vi "MultiChannelfFeedbackCooling (FPGA).vi"() -> ()   [LabVIEW 2014]
doc: "This VI will read single point values from 4 channels of a R Series board at a specified rate."
uses:
  <vilib>/rvi/Emulation/niFpgaGetClockAttributes.vi
  <vilib>/rvi/Emulation/niFpgaSctlEmulationGetInTimedLoop.vi
  <vilib>/rvi/Emulation/niFpgaEmulationReportErrorSimple.vi
  <vilib>/rvi/eio/common/nirviEmuTemplateMethod_errors.vi
  <vilib>/rvi/Memory/Memory_Emulation/nirvimemoryFastEmulation.vi
  <vilib>/rvi/Memory/Memory_Emulation/nirvimemoryEmulation.vi
  <vilib>/rvi/Emulation/niFpgaEmulationIsFPGAContextNoSignature.vi
  <vilib>/rvi/DataTransferAndStorage/Container/Common/niFpgaContainerGetUniqueNameForEmu.vi
  <vilib>/rvi/Emulation/niFpgaProcessEmulError.vi
  <vilib>/rvi/errors/nirviReportUnexpectedCaseInternalError (U32).vi
  <vilib>/rvi/Memory/Memory_Emulation/niFpgaMemoryEmulationCacheClearOnFirstRun.vi
  <vilib>/rvi/Memory/Memory_Emulation/nirvimemoryEmulationManagerCache_MakeExclusive.vi
  <vilib>/rvi/Memory/Memory_Emulation/niFpgaMemoryEmulationValidateCache.vi
  <vilib>/rvi/Memory/Memory_Emulation/nirvimemoryEmulationManagerCache_InsertValue.vi
  <vilib>/Utility/error.llb/Clear Errors.vi
  <vilib>/rvi/Memory/Memory_Emulation/nirvimemoryEmulationManagerCache_ReleaseExclusive.vi
  <vilib>/rvi/Memory/Memory_Emulation/nirvimemoryEmulationManagerCache_GetValue.vi
  <vilib>/rvi/Memory/Memory_Emulation/nirvimemoryEmulationManagerCache_SetValue.vi
  <vilib>/rvi/Emulation/niFpgaSctlEmulationResourceMgr.vi
  <vilib>/rvi/Emulation/niFpgaCriticalErrorInLSC.vi
  <vilib>/eio/EIONode/EIONode.xnode
  <vilib>/rvi/DataTransferAndStorage/Container/XNode/niFpgaContainer.xnode
  <vilib>/rvi/FXPMathLib/FxpInterpret/XNode/nifxpmath_Interpret.xnode
panel:
  in  "Piezo Z":i16
  in  "Ref AOM Lvl":i16
  in  "pg_img":fxp<+/-,24,12>
  in  "dg_img":fxp<+/-,24,12>
  in  "ig_img":fxp<+/-,24,6>
  in  "setpt_img":i16
  out "AI_img":i16
  in  "lp coeff_img":i32[](array[numeric])=[1008310688, 32715568]
  in  "Upper lim_img":fxp<+/-,16,16>
  in  "Lower lim_img":fxp<+/-,16,16>
  in  "lp coeff d2":i32[](array[numeric])=[1008310688, 32715568]
  in  "hp coeff_img":i32[](array[numeric])=[946630756, 1010186290]
  out "tot_fb_img":i16
  out "fb_img":i16
  in  "output offset_img":i16
  in  "lp coeff 2":i32[](array[numeric])=[1008310688, 32715568]
  in  "data_buffer3":i16
  in  "Arb gain (ch2)":fxp<+/-,24,12>=0.5 caption="RMS"
  in  "lp coeff 0":i32[](array[numeric])=[1008310688, 32715568]
  in  "lp coeff 1":i32[](array[numeric])=[1008310688, 32715568]
  in  "hp coeff d2":i32[](array[numeric])=[946630756, 1010186290]
  in  "hp coeff 2":i32[](array[numeric])=[946630756, 1010186290]
  in  "hp coeff 1":i32[](array[numeric])=[946630756, 1010186290]
  in  "hp coeff 0":i32[](array[numeric])=[946630756, 1010186290]
  in  "Use_PID2_X 2":bool
  out "AI5":i16
  in  "Dc Pos d2":i16
  out "tot_fb_2":i16
  out "tot_fb_1":i16
  out "tot_fb_0":i16
  out "fb_d2":i16
  in  "output offset 2":i16
  in  "output offset 1":i16
  in  "output offset 0":i16
  in  "Lower lim 4":fxp<+/-,16,16>
  in  "Upper lim d0 3":fxp<+/-,16,16>
  in  "pg d0 3":fxp<+/-,24,12>
  in  "ig d03":fxp<+/-,24,6>
  in  "dg d0 3":fxp<+/-,24,12>
  out "fb_2":i16
  in  "ig 3":fxp<+/-,24,6>
  out "written_address":u32
  in  "ready_to_write":bool
  in  "Arb steps per cycle":u16
  in  "data_buffer2":i16
  in  "data_buffer_1":i16
  in  "write_address":u16
  in  "Arb gain (ch1)":fxp<+/-,24,12>=0.5 caption="RMS"
  in  "Arb gain (ch0)":fxp<+/-,24,12>=0.5 caption="RMS"
  out "fb_1":i16
  out "fb_0":i16
  in  "Dc Pos 1":i16
  in  "Dc Pos 0":i16
  in  "Lower lim 2":fxp<+/-,16,16>
  in  "Upper lim 2":fxp<+/-,16,16>
  in  "dg 2":fxp<+/-,24,12>
  in  "pg 2":fxp<+/-,24,12>
  out "AI2":i16
  in  "Dc Pos 2":i16
  out "AI1":i16
  in  "dg 1":fxp<+/-,24,12>
  in  "Upper lim 1":fxp<+/-,16,16>
  in  "Lower lim 1":fxp<+/-,16,16>
  out "AI0":i16
  in  "dg 0":fxp<+/-,24,12>
  in  "Upper lim 0":fxp<+/-,16,16>
  in  "Lower lim 0":fxp<+/-,16,16>
  in  "Count(uSec)":u32
  out "FPGA Error Out":errorcluster
  in  "Stop":bool
  # "test"
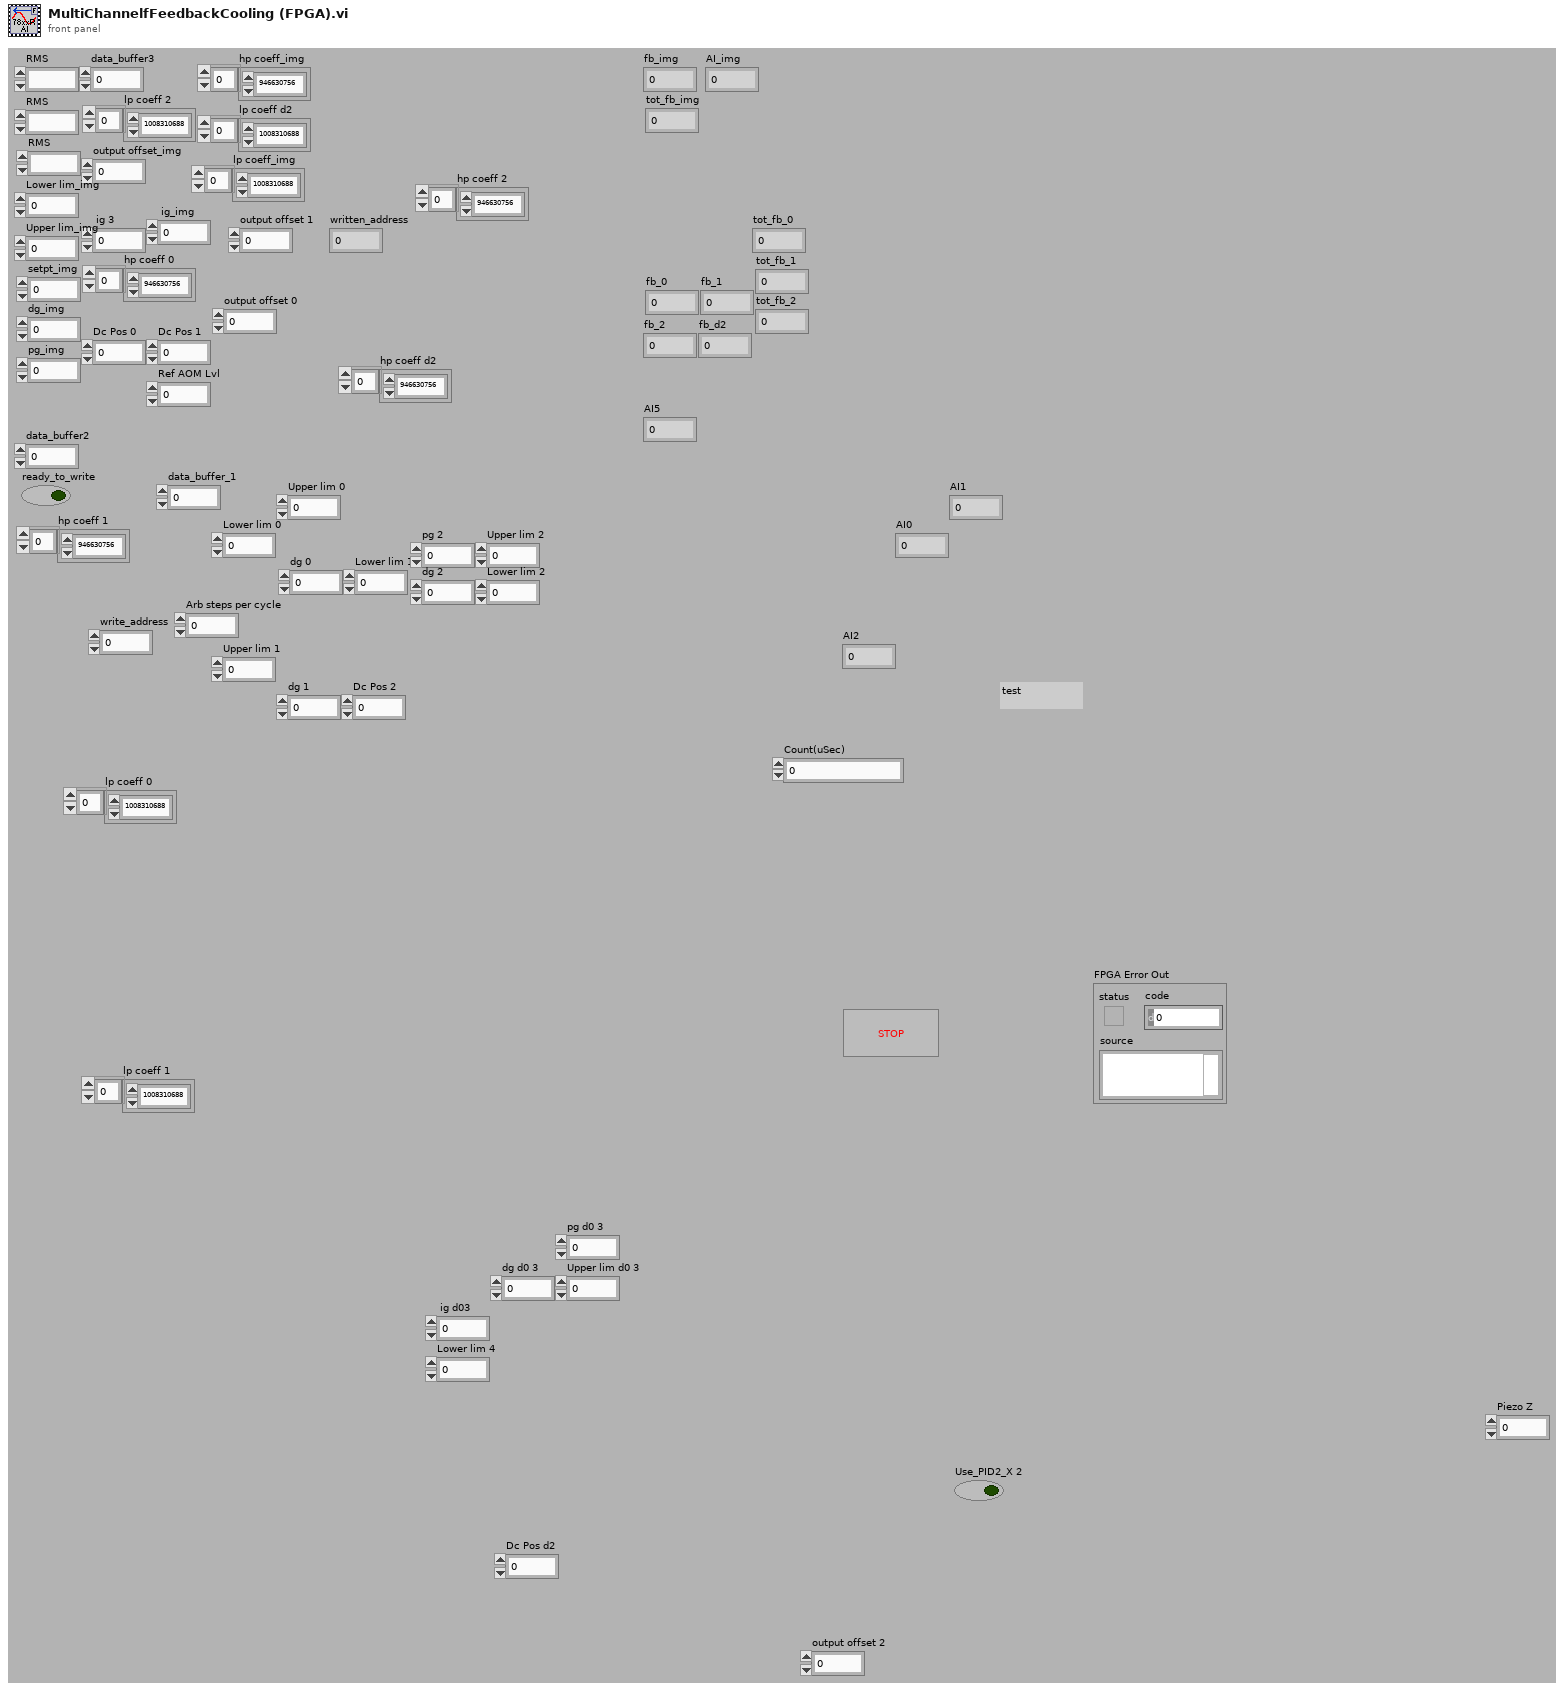
[diagram p1: front panel]
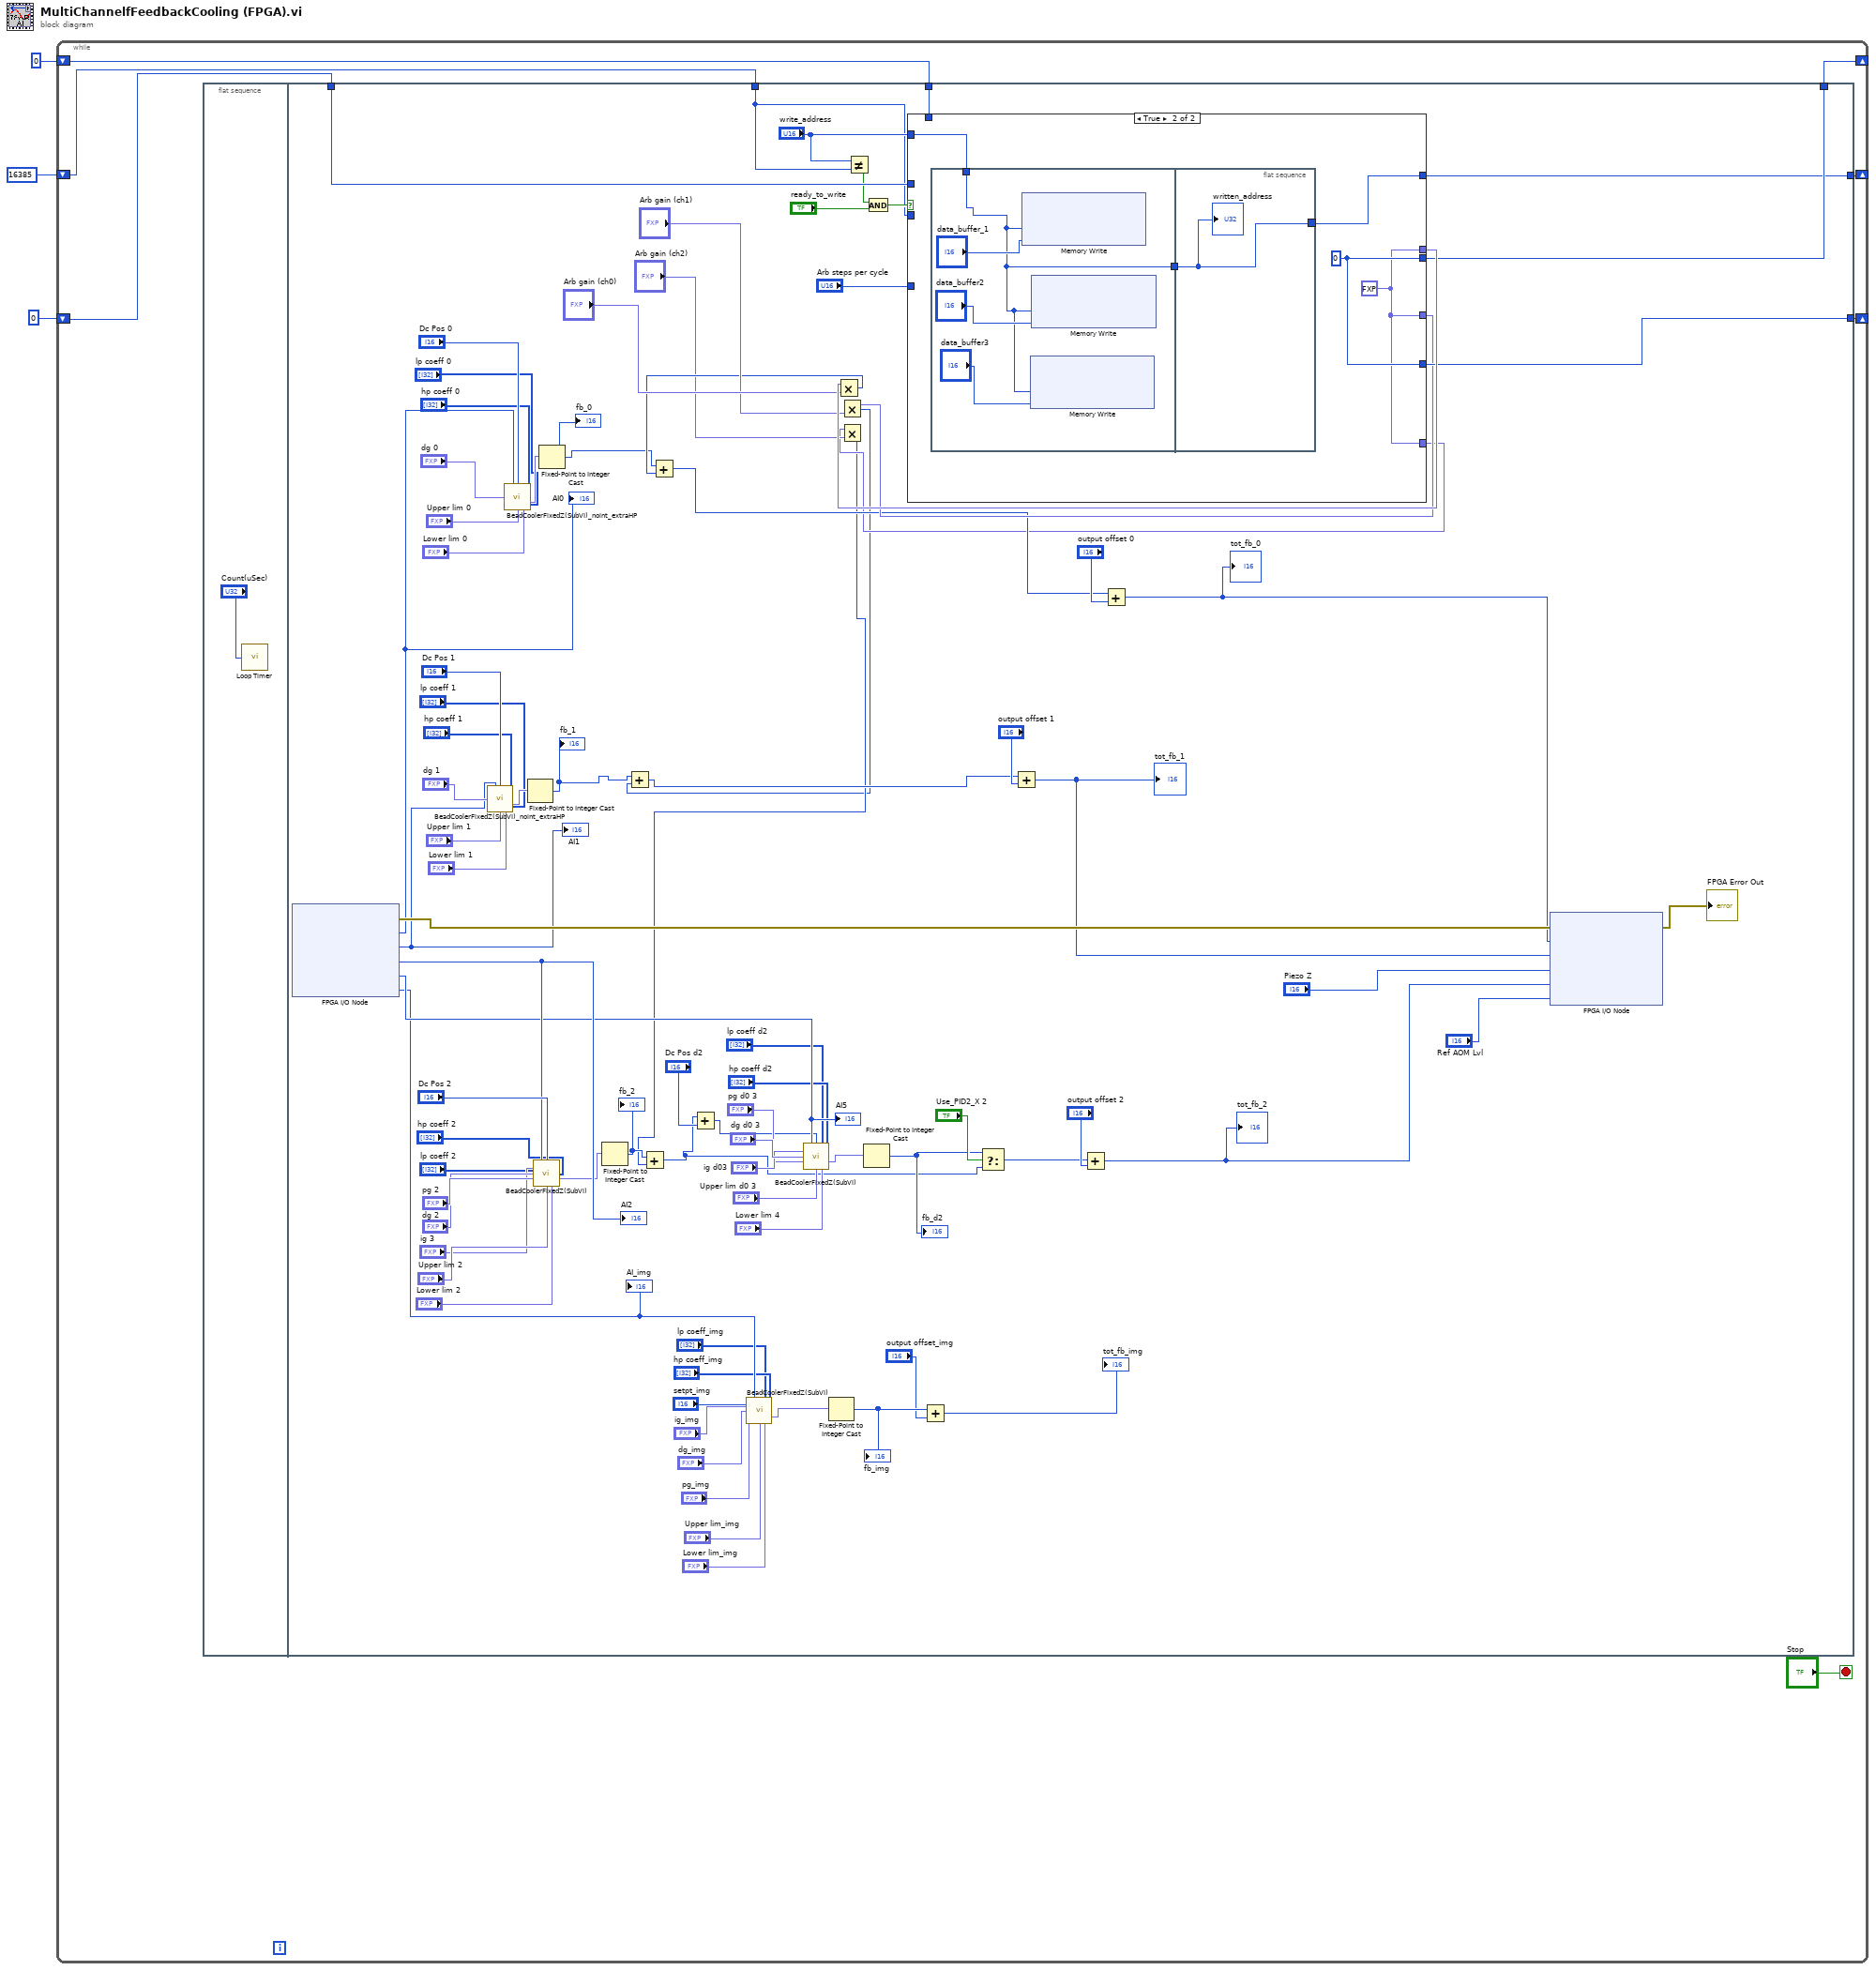
[diagram p0: block diagram]
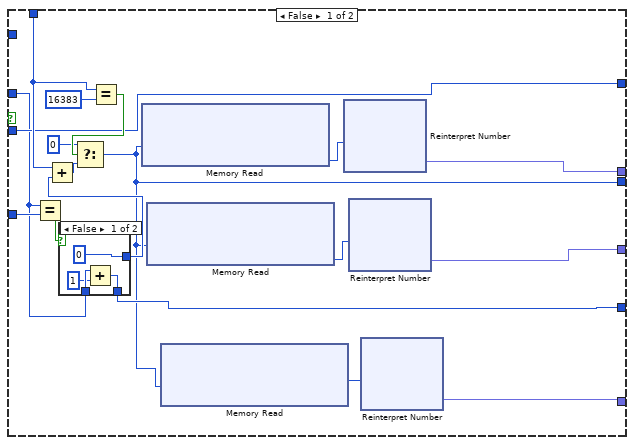
[diagram p2: hidden frame]
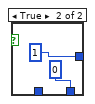
[diagram p3: hidden frame]
diagram:
  n1 = while {
    shift-right: [w9] -> _
    shift-left: u16 0 ("t") -> [w8]
    shift-right: [w7] -> _
    shift-left: u16 0 ("t") -> [w4]
    shift-right: [w6] -> _
    shift-left: u32 16385 ("write_address") -> [w5]
    stop <- "Stop" stop-if-true
    n2 = flat-sequence {
      tunnel: [w83] -> w9
      tunnel: w8 -> [w82]
      tunnel: [w80] -> w7
      tunnel: w4 -> [w79]
      tunnel: [w78] -> w6
      tunnel: w5 -> [w70]
      frame #0 {
        n3 = call "Loop Timer"("Count(uSec)"="Count(uSec)") -> ()  [unwired: 1 out]
      }
      frame #1 {
        n4 = xnode "FPGA I/O Node"() -> ("error out"=w100:errorcluster, "AI0"=w69:i16, "Connector0/AI1"=w68:i16, "Connector0/AI2"=w65:i16, "Connector0/AI5"=w53:i16, "Connector0/AI4"=w28:i16)  [unwired: 6 in, 5 out]
        "AI0" <- w69
        "AI1" <- w68
        "AI2" <- w65
        "AI5" <- w53
        "AI_img" <- w28
        n5 = call "BeadCoolerFixedZ(SubVI)_noint_extraHP.vi"("AI0"=w68, "Dc Pos"="Dc Pos 1", "dg"="dg 1", "hp coeff"="hp coeff 1", "lp coeff"="lp coeff 1", "Upper lim"="Upper lim 1", "Lower lim"="Lower lim 1") -> ("Output"=w67:fxp<+/-,16,16>)  [unwired: 8 in]
        n6 = call "BeadCoolerFixedZ(SubVI)_noint_extraHP.vi"("AI0"=w69, "Dc Pos"="Dc Pos 0", "dg"="dg 0", "hp coeff"="hp coeff 0", "lp coeff"="lp coeff 0", "Upper lim"="Upper lim 0", "Lower lim"="Lower lim 0") -> ("Output"=w71:fxp<+/-,16,16>)  [unwired: 8 in]
        n7 = Fixed-Point to Integer Cast(1:w67) -> (0:w33:i16)
        "fb_1" <- w33
        n8 = call "BeadCoolerFixedZ(SubVI).vi"("AI0"=w65, "Dc Pos"="Dc Pos 2", "lp coeff"="lp coeff 2", "ig"="ig 3", "dg"="dg 2", "hp coeff"="hp coeff 2", "pg"="pg 2", "Upper lim"="Upper lim 2", "Lower lim"="Lower lim 2") -> ("Output"=w42:fxp<+/-,16,16>)  [unwired: 6 in]
        n9 = Fixed-Point to Integer Cast(1:w71) -> (0:w36:i16)
        "fb_0" <- w36
        n10 = Fixed-Point to Integer Cast(1:w42) -> (0:w37:i16)
        "fb_2" <- w37
        n11 = call "BeadCoolerFixedZ(SubVI).vi"("AI0"=w28, "Dc Pos"="setpt_img", "lp coeff"="lp coeff_img", "ig"="ig_img", "dg"="dg_img", "hp coeff"="hp coeff_img", "pg"="pg_img", "Upper lim"="Upper lim_img", "Lower lim"="Lower lim_img") -> ("Output"=w27:fxp<+/-,16,16>)  [unwired: 6 in]
        n12 = Fixed-Point to Integer Cast(1:w27) -> (0:w26:i16)
        "fb_img" <- w26
        n13 = Not Equal?(x="write_address", y=w70) -> (x != y?=w75:bool)
        n14 = And(x=w75, y="ready_to_write") -> (x .and. y?=w76:bool)
        n15 = case shown="True" w76 {
          tunnel: [w117 w125] -> w85
          tunnel: [w102 w129] -> w83
          tunnel: w82 -> [w110 _]
          tunnel: [w111 w125] -> w73
          tunnel: "Arb steps per cycle" -> [w109 _]
          tunnel: [w104 w129] -> w80
          tunnel: w79 -> [w105 _]
          tunnel: [w108 w127] -> w78
          tunnel: w70 -> [w108 _]
          tunnel: "write_address" -> [_ w126]
          tunnel: [w101 w125] -> w34
          frame False {
            n16 = Equal?(x=w105, y=w109) -> (x = y?=w107:bool)
            n17 = case shown="False" w107 {
              tunnel: [u16 0 ("y") u16 1 ("y")] -> w106
              tunnel: w105 -> [w121 _]
              tunnel: [w119 u16 0] -> w104
              frame False {
                n18 = Add(x=w121, y=u16 1) -> (x+y=w119:u16)
              }
              frame True {
              }
            }
            n19 = Add(x=w110, y=w106) -> (x+y=w113:u16)
            n20 = Equal?(x=w110, y=u16 16383) -> (x = y?=w115:bool)
            n21 = Select(t=u16 0, s=w115, f=w113) -> (s? t:f=w102:u16)
            n22 = xnode ("Memory Read")("Address"=w102) -> ("Data"=w118:i16)  [unwired: 1 in, 1 out]
            n23 = xnode ("Memory Read")("Address"=w102) -> ("Data"=w112:i16)  [unwired: 1 in, 1 out]
            n24 = xnode ("Memory Read")("Address"=w102) -> ("Data"=w103:i16)  [unwired: 1 in, 1 out]
            n25 = xnode "Reinterpret Number"("x"=w118) -> ("y"=w117:fxp<+/-,16,16>)
            n26 = xnode "Reinterpret Number"("x"=w112) -> ("y"=w111:fxp<+/-,16,16>)
            n27 = xnode "Reinterpret Number"("x"=w103) -> ("y"=w101:fxp<+/-,16,16>)
          }
          frame True {
            w129 = u16 0
            w125 = fxp<+/-,16,16> 0.0 ("y")
            n28 = flat-sequence {
              tunnel: [w131] -> w128
              tunnel: w126 -> [w131]
              tunnel: w128 -> [w134]
              tunnel: [w134] -> w127
              frame #0 {
                n29 = xnode ("Memory Write")("Address"=w131, "Data"="data_buffer_1") -> ()  [unwired: 1 in, 1 out]
                n30 = xnode ("Memory Write")("Address"=w131, "Data"="data_buffer3") -> ()  [unwired: 1 in, 1 out]
                n31 = xnode ("Memory Write")("Address"=w131, "Data"="data_buffer2") -> ()  [unwired: 1 in, 1 out]
              }
              frame #1 {
                "written_address" <- w134
              }
            }
          }
        }
        n32 = Multiply(x=w85, y="Arb gain (ch0)") -> (x*y=w57:i16)
        n33 = Add(x=w36, y=w57) -> (x+y=w47:i16)
        n34 = Multiply(x=w73, y="Arb gain (ch1)") -> (x*y=w30:i16)
        n35 = Add(x=w33, y=w30) -> (x+y=w32:i16)
        n36 = Multiply(x=w34, y="Arb gain (ch2)") -> (x*y=w31:i16)
        n37 = Add(x=w37, y=w31) -> (x+y=w41:i16)
        n38 = Add(x=w41, y="Dc Pos d2") -> (x+y=w38:i16)
        n39 = call "BeadCoolerFixedZ(SubVI).vi"("AI0"=w53, "Dc Pos"=w38, "lp coeff"="lp coeff d2", "ig"="ig d03", "dg"="dg d0 3", "hp coeff"="hp coeff d2", "pg"="pg d0 3", "Upper lim"="Upper lim d0 3", "Lower lim"="Lower lim 4") -> ("Output"=w59:fxp<+/-,16,16>)  [unwired: 6 in]
        n40 = Fixed-Point to Integer Cast(1:w59) -> (0:w49:i16)
        "fb_d2" <- w49
        n41 = Add(x=w26, y="output offset_img") -> (x+y=→"tot_fb_img":i16)
        n42 = Select(t=w49, s="Use_PID2_X 2", f=w41) -> (s? t:f=w48:i16)
        n43 = Add(x=w32, y="output offset 1") -> (x+y=w50:i16)
        "tot_fb_1" <- w50
        n44 = Add(x=w48, y="output offset 2") -> (x+y=w13:i16)
        "tot_fb_2" <- w13
        n45 = Add(x=w47, y="output offset 0") -> (x+y=w51:i16)
        "tot_fb_0" <- w51
        n46 = xnode "FPGA I/O Node"("error in"=w100, "Connector0/AO0"=w51, "Connector0/AO1"=w50, "Connector0/AO2"="Piezo Z", "Connector0/AO3"=w13, "Connector0/AO4"="Ref AOM Lvl") -> ("error out"=→"FPGA Error Out":errorcluster)  [unwired: 5 in, 5 out]
      }
    }
  }
